vi "Untitled 4 (SubVI).vi"(8 "error in (no error)":errorcluster, 11 "Data Cluster":T1 {"Flexi-Flow Devices"."Control State"."Control Mode" items=["Bus/RS232"=0, "FLOW-BUS slave"=2, "Valve close"=3, "Controller idle"=4, "Setpoint 100%"=7, "Valve fully open"=8, "Calibration mode"=9, "Setpoint 0%"=12, "RS232"=18, "Valve steering"=20, "Valve safe state"=22]}) -> (0 "error out":errorcluster, 1 "Array":sgl[](array[numeric]), 2 "Data Table":map{string, dbl}(c390), 3 "Array 2":T3[](array[typedef]) {"Control State"."Control Mode" items=["Bus/RS232"=0, "FLOW-BUS slave"=2, "Valve close"=3, "Controller idle"=4, "Setpoint 100%"=7, "Valve fully open"=8, "Calibration mode"=9, "Setpoint 0%"=12, "RS232"=18, "Valve steering"=20, "Valve safe state"=22]})   [LabVIEW 2025, in "FlexiFlowInterface.lvlib"]
uses:
  FlexiFlowInterface/FlexiFlowInterface.lvlib
  phlair-shared-libraries/Modbus Flexi-Flow API/Control Function Values--enum.ctl
  phlair-shared-libraries/Modbus Flexi-Flow API/Bronkhorst Flexi-Flow ModbusTCP API.lvlib
  phlair-shared-libraries/Modbus Flexi-Flow API/Control Mode--enum.ctl
  FlexiFlowInterface/Modbus Flexi-Flow Controls--cluster.ctl
  FlexiFlowInterface/Modbus Flexi-Flow Measure State--cluster.ctl
  <vilib>/Plasmionique/MB Master/MB_Master_TCP/MB_Master_TCP.lvclass
  FlexiFlowInterface/Device Type--enum.ctl
  FlexiFlowInterface/Modbus Flexi-Flow State--cluster.ctl
  FlexiFlowInterface/Modbus TCP Connection Settings--cluster.ctl
  FlexiFlowInterface/Module Data--cluster.ctl
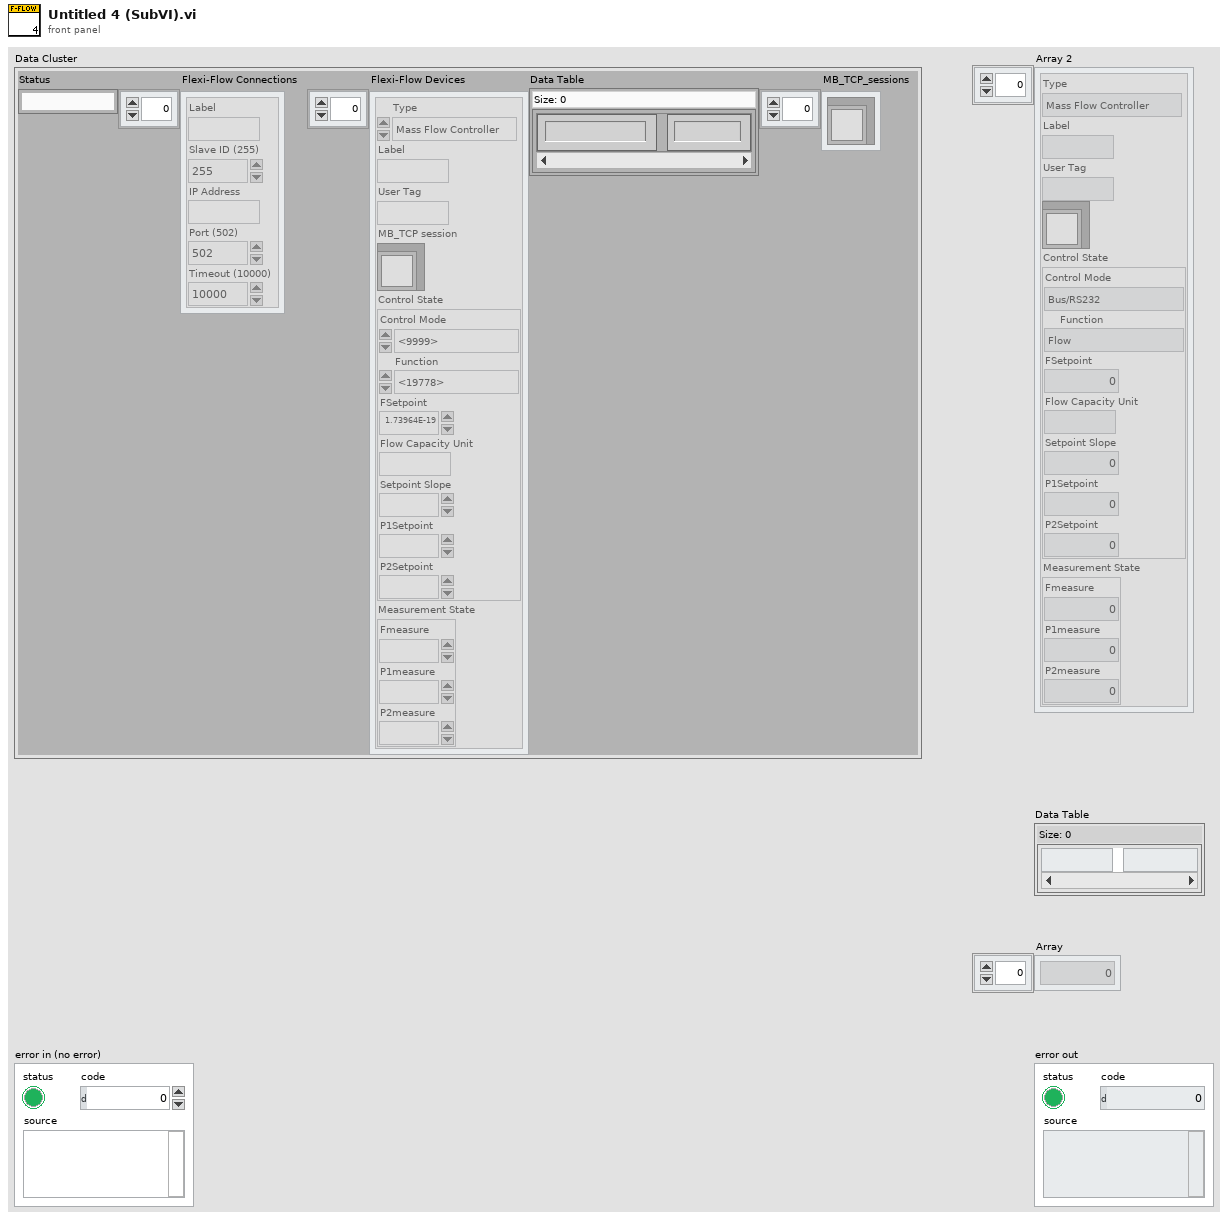
[diagram p1: front panel]
types:
  T1 = typedef "FlexiFlowInterface.lvlib/Module Data--cluster.ctl" = cluster{"Status":string, "Flexi-Flow Connections":T2[], "Flexi-Flow Devices":T3[], "Data Table":map{string, dbl}, "MB_TCP_sessions":refnum<class "MB_Master_TCP.lvclass">[]}
  T2 = typedef "FlexiFlowInterface.lvlib/Modbus TCP Connection Settings--cluster.ctl" = cluster{"Label":string, "Slave ID (255)":u8, "IP Address":string, "Port (502)":u16, "Timeout (10000)":i32}
  T3 = typedef "FlexiFlowInterface.lvlib/Modbus Flexi-Flow State--cluster.ctl" = cluster{"Type":T4, "Label":string, "User Tag":string, "MB_TCP session":refnum<class "MB_Master_TCP.lvclass">, "Control State":T5, "Measurement State":T8}
  T4 = typedef "Device Type--enum.ctl" = enum16{"Mass Flow Controller", "Mass Flow Meter"}
  T5 = typedef "FlexiFlowInterface.lvlib/Modbus Flexi-Flow Controls--cluster.ctl" = cluster{"Control Mode":T6, "Function":T7, "FSetpoint":sgl, "Flow Capacity Unit":string, "Setpoint Slope":u16, "P1Setpoint":sgl, "P2Setpoint":sgl}
  T6 = typedef "Bronkhorst Flexi-Flow ModbusTCP API.lvlib/Control Mode--enum.ctl" = u16
  T7 = typedef "Bronkhorst Flexi-Flow ModbusTCP API.lvlib/Control Function Values--enum.ctl" = enum16{"Flow", "Upstream pressure", "Downstream pressure", "Flow with upstream pressure limit", "Flow with downstream pressure limit", "Upstream pressure with flow limit", "Downstream pressure with flow limit"}
  T8 = typedef "FlexiFlowInterface.lvlib/Modbus Flexi-Flow Measure State--cluster.ctl" = cluster{"Fmeasure":dbl, "P1measure":sgl, "P2measure":sgl}
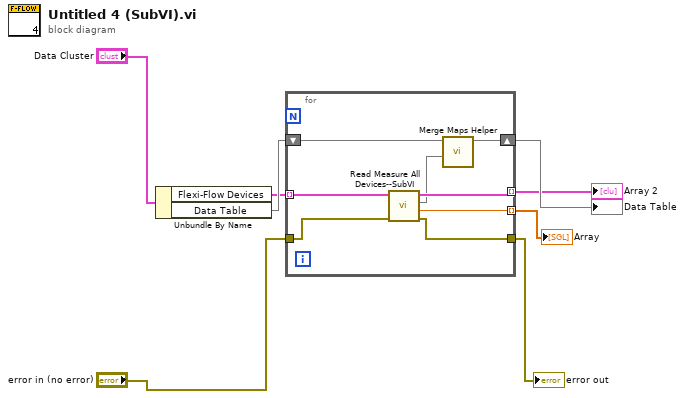
[diagram p0: block diagram]
diagram:
  n1 = Unbundle By Name("Data Cluster") -> ("Flexi-Flow Devices"=w2:T3[], "Data Table"=w5:map{string, dbl})
  n2 = for {
    tunnel: w2 -> [w13] mode=indexing
    tunnel: [w14] -> w4 mode=indexing
    tunnel: "error in (no error)" -> [w16]
    tunnel: [w15] -> w8
    shift-right: [w11] -> w6
    shift-left: w5 -> [w12]
    tunnel: [w9] -> w7 mode=indexing
    n3 = call "Read Measure All Devices--SubVI.vi"("error in (no error)"=w16, "Flexi-Flow in"=w13) -> ("error out"=w15:errorcluster, "Value"=w9:sgl, "map out"=w10:map{string, dbl}, "Flexi-Flow out"=w14:T3)  [unwired: 6 in]
    n4 = call "Merge Maps Helper.vi"("map in"=w10, "Data Table in"=w12) -> ("Data Table out"=w11:map{string, dbl})  [unwired: 9 in]
  }
  "error out" <- w8
  "Array" <- w7
  "Data Table" <- w6
  "Array 2" <- w4
